vi "Actor Core.vi"(8 "error in":errorcluster, 11 "Cooler Panel in":refnum<class "Cooler Panel.lvclass">) -> (0 "error out":errorcluster, 3 "Actor out":refnum<class "Actor.lvclass">)   [LabVIEW 2012, in "Cooler UI.lvlib" / "Cooler Panel.lvclass"]
doc: "(<B>Filename</B>: Actor Framework.lvlib:Actor.lvclass:Actor Core.vi)\n\nReceives messages to the actor, reacts to them, and initiates any error handling that may shut the actor down.\n\nDescendant classes may override this VI to append parallel tasks for the actor to complete while it handles messages. Overrides use the Call Parent Method node."
uses:
  Cooler Panel.lvclass
  <vilib>/ActorFramework/Actor/Actor.lvclass
  Cooler UI with Events/Cooler UI with Events.lvclass/Cooler UI with Events.ctl
  Cooler UI with Events/Cooler UI with Events.lvclass
  <vilib>/ActorFramework/Actor/Actor.lvclass/Actor.ctl
  <vilib>/ActorFramework/Message Enqueuer/Message Enqueuer.lvclass/Message Enqueuer.ctl
  Cooler UI with Events Messages/Update Temperature Msg/Update Temperature Msg.lvclass/Update Temperature Msg.ctl
  <vilib>/ActorFramework/Message Enqueuer/Init from Existing Queue.vi
  <vilib>/ActorFramework/Message Enqueuer/Enqueue.vi
  <vilib>/ActorFramework/Message Priority Queue/Priority Enqueue.vi
  <vilib>/ActorFramework/Message Enqueuer/Message Enqueuer.lvclass
  Cooler UI with Events Messages/Update Temperature Msg/Update Temperature Msg.lvclass
panel:
  out "Pump":bool
  out "Temperature":dbl(slide) scale=0.0..120.0
  out "Fan A":bool
  out "Fan B":bool
  out "Fault A":bool
  out "Fault B":bool
  in  "Desired Temperature":dbl=75.0
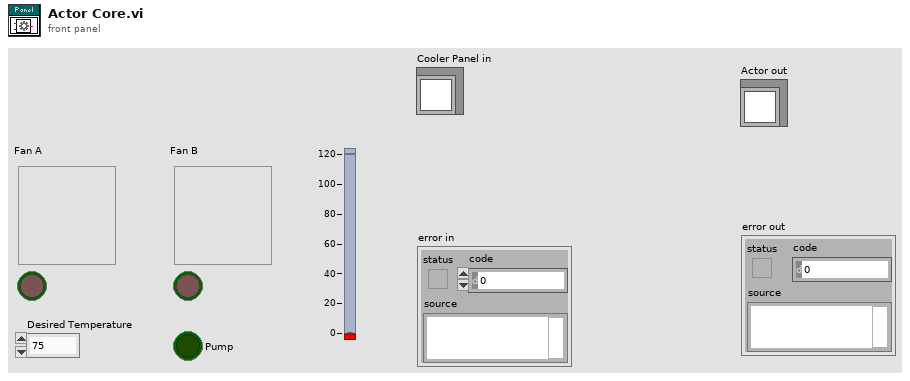
[diagram p1: front panel]
types:
  T1 = enum32{"Invalid", "Standard", "Closed", "Hidden", "Minimized", "Maximized"}
  T2 = typedef "Cooler UI.lvlib/Cooler UI with Events.lvclass/Events.ctl" = cluster{"Fan Status":refnum<user-event>, "Temperature":refnum<user-event>, "Pump":refnum<user-event>}
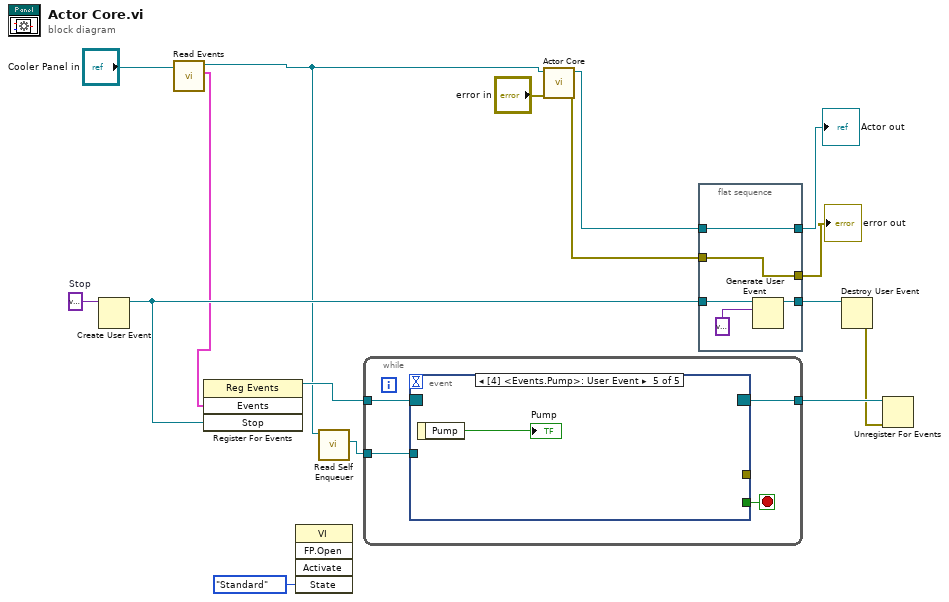
[diagram p0: block diagram]
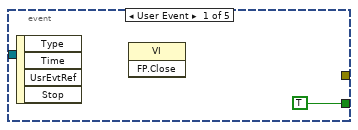
[diagram p2: hidden frame]
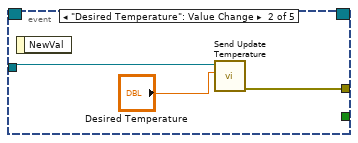
[diagram p3: hidden frame]
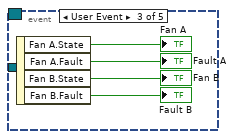
[diagram p4: hidden frame]
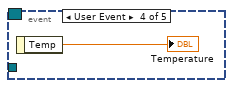
[diagram p5: hidden frame]
diagram:
  w14 = variant  # Stop
  n1 = Create User Event(user event datatype=w14) -> (user event=w9:refnum<user-event>)  [unwired: 1 in, 1 out]
  n2 = call "Read Events.vi"("Cooler UI with Events in"="Cooler Panel in") -> ("Events"=w7:T2, "Cooler UI with Events out"=w6:refnum<class "Cooler Panel.lvclass">)  [unwired: 9 in]
  n3 = register-events(w7, w9) -> (reference out=w15:refnum<event-registration>)  [unwired: 2 in, 1 out]
  n4 = invoke class="VI" method="FP.Open"("State"=T1."Standard") -> ()  [unwired: 4 in, 5 out]
  n5 = call <vilib>:"Read Self Enqueuer.vi"("Actor"=w6) -> ("Self Enqueuer"=w5:refnum<class "Message Enqueuer.lvclass">)  [unwired: 10 in]
  n6 = while {
    tunnel: w15 -> [w20]
    tunnel: [w19] -> w13
    tunnel: w5 -> [w17]
    stop <- w18 stop-if-true
    n7 = event shown="[4] <Events.Pump>: User Event" {
      selector: w20 -> [_ _ _ _ _]
      dyn-events: [_ _ _ _ _] -> w19
      timeout: _ -> [_ _ _ _ _]
      tunnel: [TRUE _ _ _ _] -> w18
      tunnel: w17 -> [_ w23 _ _ _]
      tunnel: [_ w22 _ _ _] -> _
      event User Event {
        n8 = event-data() -> ()  [unwired: 1 in, 4 out]
        n9 = invoke class="VI" method="FP.Close"() -> ()  [unwired: 3 in, 3 out]
      }
      event "Desired Temperature": Value Change {
        n10 = event-data() -> ()  [unwired: 1 in, 1 out]
        n11 = call "Send Update Temperature.vi"("Temperature"="Desired Temperature", "Message Enqueuer"=w23) -> ("error out"=w22:errorcluster)  [unwired: 8 in, 1 out]
      }
      event User Event {
        n12 = event-data() -> ("Fan A.State"=→"Fan A":bool, "Fan A.Fault"=→"Fault A":bool, "Fan B.State"=→"Fan B":bool, "Fan B.Fault"=→"Fault B":bool)  [unwired: 1 in]
      }
      event User Event {
        n13 = event-data() -> ("Temp"=→"Temperature":dbl)  [unwired: 1 in]
      }
      event User Event {
        n14 = event-data() -> ("Pump"=→"Pump":bool)  [unwired: 1 in]
      }
    }
  }
  n15 = call-parent "Actor Core.vi"("error in"="error in", "Actor in"=w6) -> ("error out"=w1:errorcluster, "Actor out"=w3:refnum<class "Actor.lvclass">)  [unwired: 8 in]
  n16 = flat-sequence {
    tunnel: [w35] -> w11
    tunnel: w9 -> [w34]
    tunnel: [w32] -> w4
    tunnel: w3 -> [w32]
    tunnel: [w31] -> w2
    tunnel: w1 -> [w31]
    frame #0 {
      n17 = Generate User Event(user event=w34, event data cluster=variant ("Stop")) -> (user event out=w35:refnum<user-event>)  [unwired: 1 in, 1 out]
    }
  }
  n18 = Destroy User Event(user event=w11) -> (error out=w12:errorcluster)  [unwired: 1 in]
  n19 = Unregister For Events(event registration refnum=w13, error in=w12) -> ()  [unwired: 1 out]
  "error out" <- w2
  "Actor out" <- w4
